vi "ep_Write Voltage Sensitivity.vi"(8 "error in (no error)":errorcluster, 10 "voltage sensitivity":dbl[](array[numeric]), 11 "system info in":refnum<class "EP System Info.lvclass">) -> (0 "error out":errorcluster, 3 "system info out":refnum<class "EP System Info.lvclass">)   [LabVIEW 2011, in "NI_EP_Power Quality.lvlib" / "EP System Info.lvclass"]
uses:
  <vilib>/addons/Electrical Power/PQ/Common/Classes/System Info/EP System Info.lvclass
  <vilib>/addons/Electrical Power/PQ/Common/Classes/System Info/EP System Info.lvclass/EP System Info.ctl
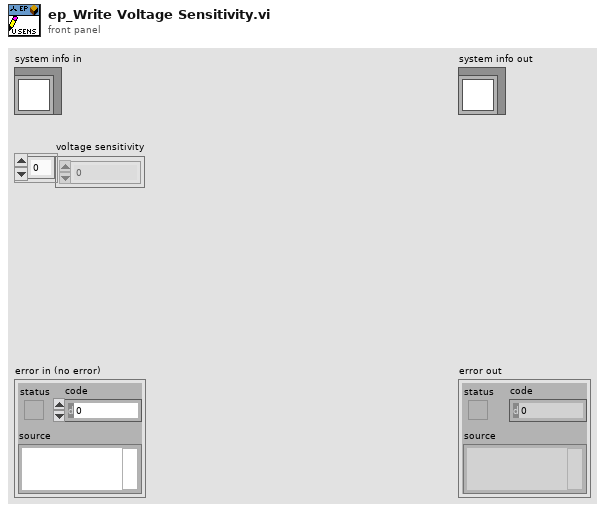
[diagram p1: front panel]
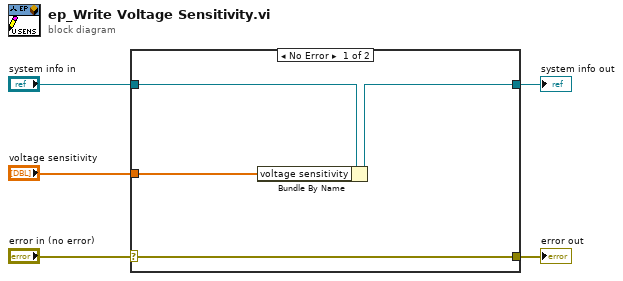
[diagram p0: block diagram]
diagram:
  n1 = case shown="No Error" "error in (no error)" {
    selector: "error in (no error)" -> [w9 w10]
    tunnel: [w9 w10] -> w4
    tunnel: [w6 w11] -> w2
    tunnel: "system info in" -> [w8 w11]
    tunnel: "voltage sensitivity" -> [w7 _]
    frame No Error {
      n2 = Bundle By Name(cluster=w8, "voltage sensitivity"=w7) -> (w6:refnum<class "EP System Info.lvclass">)
    }
    frame Error {
    }
  }
  "error out" <- w4
  "system info out" <- w2
